vi "Write_a_Decrypted_File.vi"(7 "name of Folder":string, 8 "error in (no error)":errorcluster, 9 "name of file":string, 10 "Dencrypted text":string, 11 "object in":refnum<class "Crypter.lvclass">) -> (0 "error out":errorcluster, 3 "object out":refnum<class "Crypter.lvclass">)   [LabVIEW 2016, in "Crypter.lvclass"]
uses:
  Crypter.lvclass
  Crypter.lvclass/Crypter.ctl
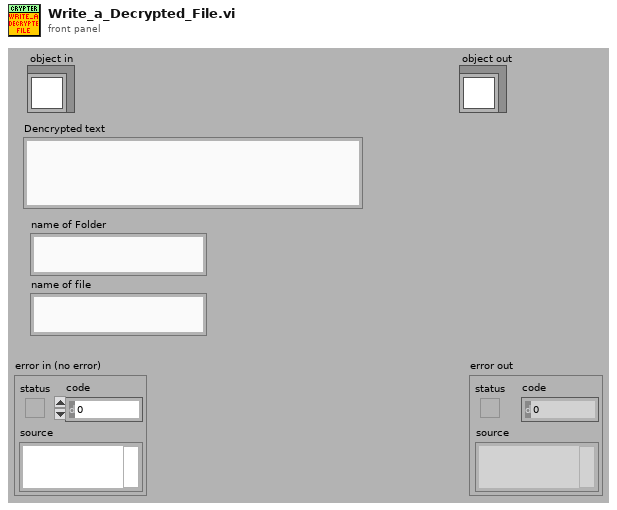
[diagram p1: front panel]
types:
  T1 = enum16{"open", "replace", "create", "open or create", "replace or create", "replace or create with confirmation"}
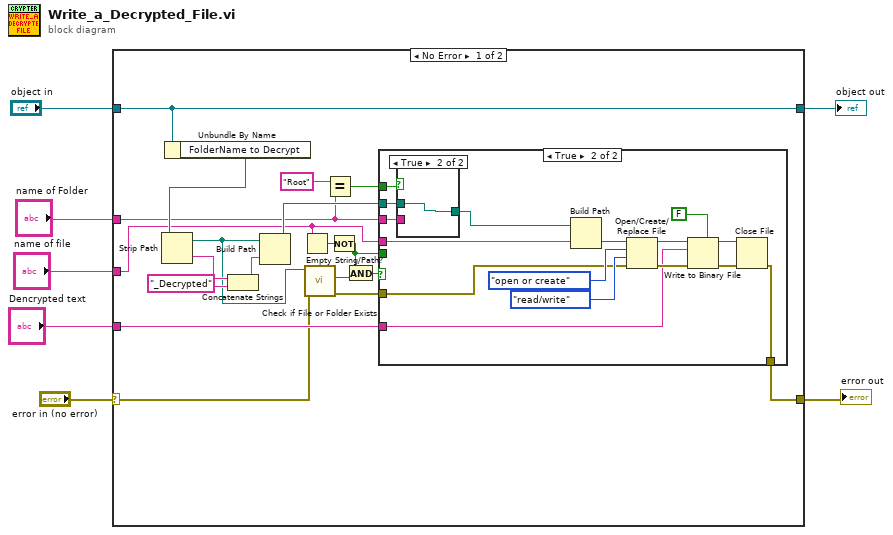
[diagram p0: block diagram]
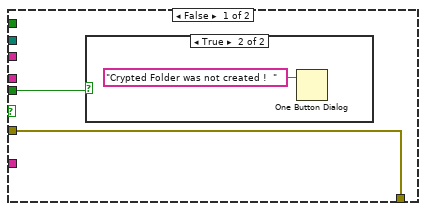
[diagram p2: hidden frame]
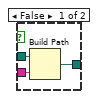
[diagram p4: hidden frame]
diagram:
  n1 = case shown="No Error" "error in (no error)" {
    selector: "error in (no error)" -> [w17 w51]
    tunnel: [w16 w51] -> w6
    tunnel: [w26 w50] -> w4
    tunnel: "object in" -> [w26 w50]
    tunnel: "name of Folder" -> [w15 _]
    tunnel: "Dencrypted text" -> [w25 _]
    tunnel: "name of file" -> [w11 _]
    frame No Error {
      n2 = Unbundle By Name(w26) -> ("FolderName to Decrypt"=w21:path)
      n3 = Strip Path(path=w21) -> (stripped path=w19:path, name=w23:string)
      n4 = Concatenate Strings(w23, "_Decrypted") -> (w22:string)
      n5 = Build Path(base path=w19, name or relative path=w22) -> (appended path=w20:path)
      n6 = Empty String/Path?(string/path=w11) -> (empty?=w10:bool)
      n7 = call <vilib>:"Check if File or Folder Exists.vi"("error in (no error)"=w17, "path"=w19) -> ("error out"=w18:errorcluster, "file or folder exists?"=w12:bool)  [unwired: 7 in, 1 out]
      n8 = Equal?(x="Root", y=w15) -> (x = y?=w13:bool)
      n9 = Not(x=w10) -> (.not. x?=w8:bool)
      n10 = And(x=w8, y=w12) -> (x .and. y?=w9:bool)
      n11 = case shown="True" w9 {
        tunnel: w15 -> [_ w39]
        tunnel: w25 -> [_ w38]
        tunnel: w20 -> [_ w37]
        tunnel: w18 -> [w28 w31]
        tunnel: [w28 w36] -> w16
        tunnel: w11 -> [_ w34]
        tunnel: w13 -> [_ w33]
        tunnel: w8 -> [w27 _]
        frame False {
          n12 = case shown="True" w27 {
            frame False {
            }
            frame True {
              n13 = One Button Dialog(message="Crypted Folder was not created !  ") -> ()  [unwired: 1 in, 1 out]
            }
          }
        }
        frame True {
          n14 = case shown="True" w33 {
            tunnel: w39 -> [w48 _]
            tunnel: w37 -> [w47 w49]
            tunnel: [w46 w49] -> w35
            frame False {
              n15 = Build Path(base path=w47, name or relative path=w48) -> (appended path=w46:path)
            }
            frame True {
            }
          }
          n16 = Build Path(base path=w35, name or relative path=w34) -> (appended path=w32:path)
          n17 = Open/Create/Replace File(file path (use dialog)=w32, error in=w31, operation (0:open)=T1."open or create", access (0:read/write)=enum16{"read/write", "read-only", "write-only"}."read/write") -> (refnum out=w43:refnum<file>, error out=w42:errorcluster)  [unwired: 2 in, 1 out]
          n18 = Write to Binary File(file (use dialog)=w43, data=w38, error in=w42, 5:FALSE ("prepend array or string size? (T)")) -> (refnum out=w40:refnum<file>, error out=w41:errorcluster)  [unwired: 2 in, 1 out]
          n19 = Close File(refnum=w40, error in=w41) -> (error out=w36:errorcluster)  [unwired: 1 out]
        }
      }
    }
    frame Error {
    }
  }
  "error out" <- w6
  "object out" <- w4
